vi "Form RMC Sentence.vi"(8 "error in (no error)":errorcluster, 11 "RMC data":T1={"time of fix"={"included?"=TRUE, "time"=timestamp(1451718000 s since 1904-01-01)}, "status"={"included?"=TRUE, "value"=0}, "latitude"={"included?"=TRUE, "latitude (deg)"=0.0}, "longitude"={"included?"=TRUE, "longitude (deg)"=0.0}, "ground speed"={"included?"=TRUE, "speed (knots)"=0.0}, "true track angle"={"included?"=TRUE, "angle (deg)"=0.0}, "magnetic variation"={"included?"=TRUE, "variation (deg)"=0.0}, "type of fix"={"included?"=TRUE, "mode"=0}} {"type of fix"."mode" items=["", "Simulator", "Not Valid", "Estimated", "Differential", "Autonomous"]; "status"."value" items=["Void", "Active"]}) -> (0 "error out":errorcluster, 3 "RMC sentence":string)   [LabVIEW 2009]
doc: "Creates an NMEA sentence using the data you specify for a particular sentence type. You must manually select the polymorphic instance to use."
uses:
  typedefs/RMC Data.ctl
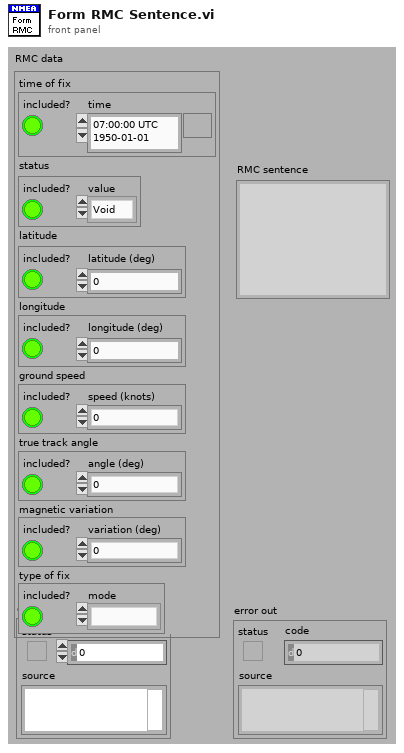
[diagram p1: front panel]
types:
  T1 = typedef "RMC Data.ctl" = cluster{"time of fix":cluster{"included?":bool, "time":timestamp}, "status":cluster{"included?":bool, "value":u16}, "latitude":cluster{"included?":bool, "latitude (deg)":dbl}, "longitude":cluster{"included?":bool, "longitude (deg)":dbl}, "ground speed":cluster{"included?":bool, "speed (knots)":dbl}, "true track angle":cluster{"included?":bool, "angle (deg)":dbl}, "magnetic variation":cluster{"included?":bool, "variation (deg)":dbl}, "type of fix":cluster{"included?":bool, "mode":u16}}
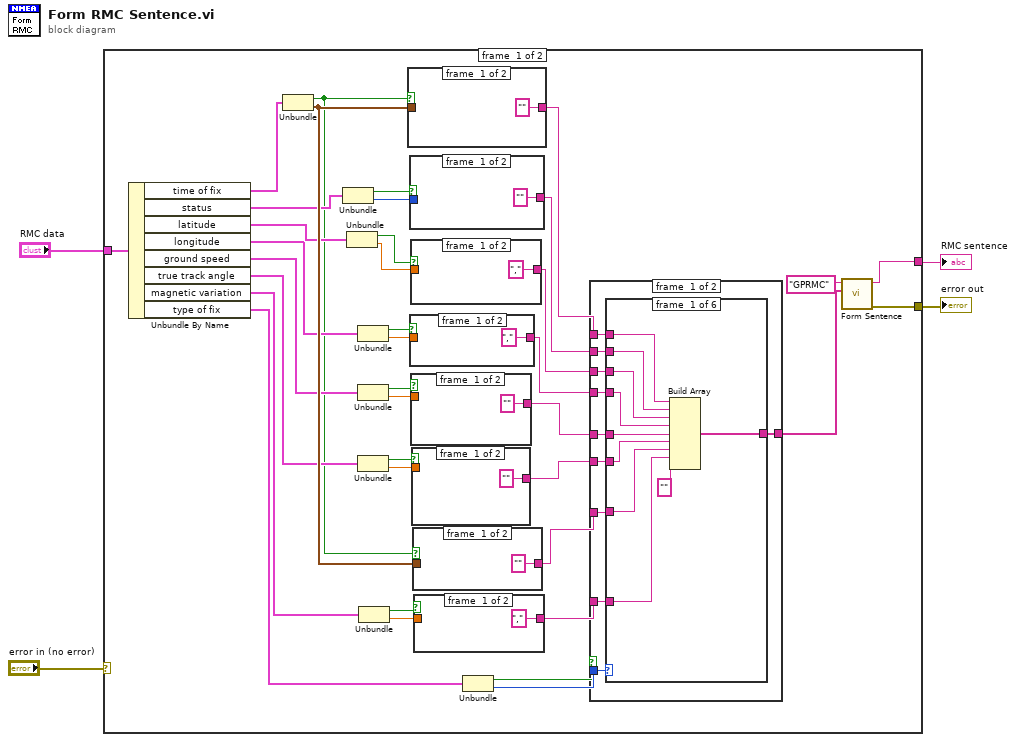
[diagram p0: block diagram]
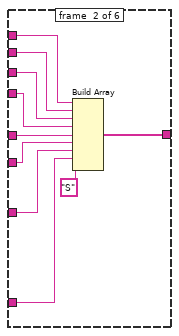
[diagram p2: hidden frame]
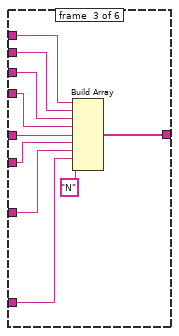
[diagram p3: hidden frame]
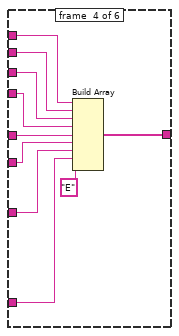
[diagram p4: hidden frame]
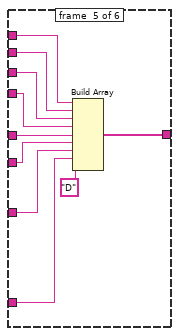
[diagram p5: hidden frame]
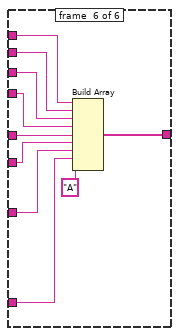
[diagram p6: hidden frame]
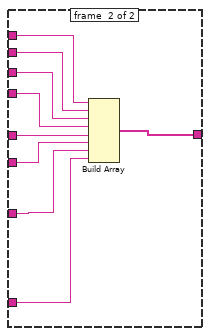
[diagram p7: hidden frame]
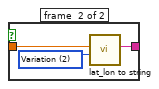
[diagram p8: hidden frame]
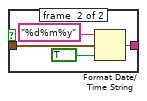
[diagram p9: hidden frame]
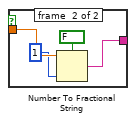
[diagram p10: hidden frame]
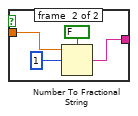
[diagram p11: hidden frame]
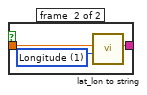
[diagram p12: hidden frame]
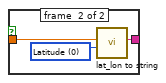
[diagram p13: hidden frame]
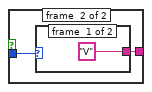
[diagram p14: hidden frame]
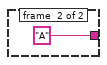
[diagram p15: hidden frame]
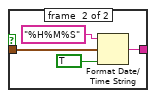
[diagram p16: hidden frame]
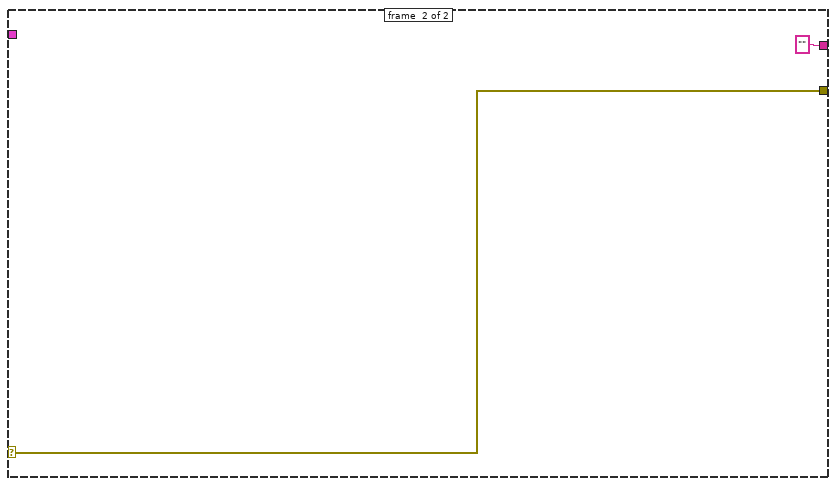
[diagram p17: hidden frame]
diagram:
  n1 = case shown="No Error" "error in (no error)" {
    selector: "error in (no error)" -> [_ w158]
    tunnel: [w40 w158] -> w3
    tunnel: [w39 "" ("NMEA Sentence")] -> w4
    tunnel: "RMC data" -> [w38 _]
    frame #0 {
      n2 = Unbundle By Name(w38) -> ("time of fix"=w28:cluster{"included?":bool, "time":timestamp}, "status"=w26:cluster{"included?":bool, "value":u16}, "latitude"=w23:cluster{"included?":bool, "latitude (deg)":dbl}, "longitude"=w21:cluster{"included?":bool, "longitude (deg)":dbl}, "ground speed"=w17:cluster{"included?":bool, "speed (knots)":dbl}, "true track angle"=w14:cluster{"included?":bool, "angle (deg)":dbl}, "magnetic variation"=w10:cluster{"included?":bool, "variation (deg)":dbl}, "type of fix"=w7:cluster{"included?":bool, "mode":u16})
      n3 = Unbundle(w28) -> ("included?"=w11:bool, "time"=w27:timestamp)
      n4 = Unbundle(w26) -> ("included?"=w24:bool, "value"=w25:u16)
      n5 = Unbundle(w23) -> ("included?"=w18:bool, "latitude (deg)"=w22:dbl)
      n6 = Unbundle(w21) -> ("included?"=w19:bool, "longitude (deg)"=w20:dbl)
      n7 = Unbundle(w17) -> ("included?"=w15:bool, "speed (knots)"=w16:dbl)
      n8 = Unbundle(w14) -> ("included?"=w12:bool, "angle (deg)"=w13:dbl)
      n9 = Unbundle(w10) -> ("included?"=w8:bool, "variation (deg)"=w9:dbl)
      n10 = case shown="True" w11 {
        tunnel: ["" ("date/time string") w156] -> w37
        tunnel: w27 -> [_ w155]
        frame #0 {
        }
        frame #1 {
          n11 = Format Date/Time String(time format string (%c)="%H%M%S", seconds (now)=w155, UTC format=TRUE) -> (date/time string=w156:string)
        }
      }
      n12 = case shown="True" w24 {
        tunnel: w25 -> [_ w150]
        tunnel: ["" w149] -> w36
        frame #0 {
        }
        frame #1 {
          n13 = case shown="1" w150 {
            tunnel: ["V" "A"] -> w149
            frame #0 {
            }
            frame #1 {
            }
          }
        }
      }
      n14 = case shown="True" w19 {
        tunnel: ["," ("NMEA String for Lat/Lon") w142] -> w34
        tunnel: w20 -> [_ w141]
        frame #0 {
        }
        frame #1 {
          w143 = u16 1 items=["Latitude", "Longitude"] ("Lat/Lon")
          n15 = call "lat_lon to string.vi"("lat/lon"=w143, "composite value"=w141) -> ("NMEA string for lat/lon"=w142:string)  [unwired: 9 out]
        }
      }
      n16 = case shown="True" w18 {
        tunnel: w22 -> [_ w147]
        tunnel: ["," ("NMEA String for Lat/Lon") w145] -> w35
        frame #0 {
        }
        frame #1 {
          w146 = u16 0 items=["Latitude", "Longitude"] ("Lat/Lon")
          n17 = call "lat_lon to string.vi"("lat/lon"=w146, "composite value"=w147) -> ("NMEA string for lat/lon"=w145:string)  [unwired: 9 out]
        }
      }
      n18 = case shown="True" w15 {
        tunnel: ["" w139] -> w33
        tunnel: w16 -> [_ w138]
        frame #0 {
        }
        frame #1 {
          n19 = Number To Fractional String(use system decimal point (T)=FALSE, number=w138, precision (6)=i16 1) -> (F-format string=w139:string)  [unwired: 1 out]
        }
      }
      n20 = case shown="True" w12 {
        tunnel: ["" w134] -> w32
        tunnel: w13 -> [_ w133]
        frame #0 {
        }
        frame #1 {
          n21 = Number To Fractional String(use system decimal point (T)=FALSE, number=w133, precision (6)=i16 1) -> (F-format string=w134:string)  [unwired: 1 out]
        }
      }
      n22 = case shown="True" w11 {
        tunnel: ["" ("date/time string") w128] -> w31
        tunnel: w27 -> [_ w127]
        frame #0 {
        }
        frame #1 {
          n23 = Format Date/Time String(time format string (%c)="%d%m%y", seconds (now)=w127, UTC format=TRUE) -> (date/time string=w128:string)
        }
      }
      n24 = case shown="True" w8 {
        tunnel: ["," ("NMEA String for Lat/Lon") w124] -> w30
        tunnel: w9 -> [_ w123]
        frame #0 {
        }
        frame #1 {
          w122 = u16 2 items=["Latitude", "Longitude", "Variation"] ("Lat/Lon")
          n25 = call "lat_lon to string.vi"("lat/lon"=w122, "composite value"=w123) -> ("NMEA string for lat/lon"=w124:string)  [unwired: 9 out]
        }
      }
      n26 = Unbundle(w7) -> ("included?"=w5:bool, "mode"=w6:u16)
      n27 = case shown="True" w5 {
        tunnel: w37 -> [w51 w120]
        tunnel: w36 -> [w50 w119]
        tunnel: w35 -> [w49 w118]
        tunnel: w34 -> [w48 w117]
        tunnel: w33 -> [w47 w116]
        tunnel: w32 -> [w46 w115]
        tunnel: w31 -> [w45 w114]
        tunnel: w30 -> [w44 w113]
        tunnel: [w43 w112] -> w29
        tunnel: w6 -> [w42 _]
        frame #0 {
          n28 = case shown="Default" w42 {
            tunnel: w51 -> [w61 w71 w81 w91 w101 w111]
            tunnel: w50 -> [w60 w70 w80 w90 w100 w110]
            tunnel: w49 -> [w59 w69 w79 w89 w99 w109]
            tunnel: w48 -> [w58 w68 w78 w88 w98 w108]
            tunnel: w47 -> [w57 w67 w77 w87 w97 w107]
            tunnel: w46 -> [w56 w66 w76 w86 w96 w106]
            tunnel: w45 -> [w55 w65 w75 w85 w95 w105]
            tunnel: w44 -> [w54 w64 w74 w84 w94 w104]
            tunnel: [w53 w63 w73 w83 w93 w103] -> w43
            frame #0 {
              n29 = Build Array(w61, w60, w59, w58, w57, w56, w55, w54, "" ("element")) -> (w53:string[])
            }
            frame #1 {
              n30 = Build Array(w71, w70, w69, w68, w67, w66, w65, w64, "S" ("element")) -> (w63:string[])
            }
            frame #2 {
              n31 = Build Array(w81, w80, w79, w78, w77, w76, w75, w74, "N" ("element")) -> (w73:string[])
            }
            frame #3 {
              n32 = Build Array(w91, w90, w89, w88, w87, w86, w85, w84, "E" ("element")) -> (w83:string[])
            }
            frame #4 {
              n33 = Build Array(w101, w100, w99, w98, w97, w96, w95, w94, "D" ("element")) -> (w93:string[])
            }
            frame #5 {
              n34 = Build Array(w111, w110, w109, w108, w107, w106, w105, w104, "A" ("element")) -> (w103:string[])
            }
          }
        }
        frame #1 {
          n35 = Build Array(w120, w119, w118, w117, w116, w115, w114, w113) -> (w112:string[])
        }
      }
      n36 = call "Form Sentence.vi"("sentence data"=w29, "sentence type"="GPRMC" ("Sentence Type")) -> ("error out"=w40:errorcluster, "sentence"=w39:string)  [unwired: 6 in]
    }
    frame #1 {
    }
  }
  "error out" <- w3
  "RMC sentence" <- w4
